vi "iHR550 Correct Center.vi"(1 "Set?":bool=TRUE, 2 "Grating Index":i32=1, 3 "Position In (nm)":dbl=897.9988) -> (0 "Position Out (nm)":dbl=897.9988)   [LabVIEW 2010]
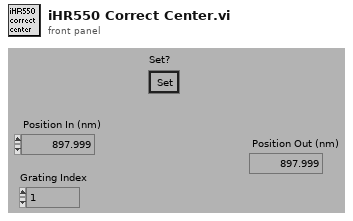
[diagram p1: front panel]
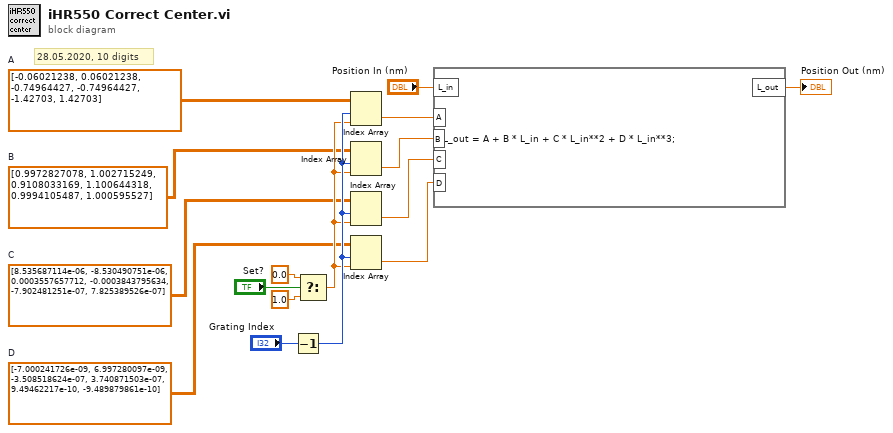
[diagram p0: block diagram]
diagram:
  w1 = dbl[][] [[-7.000241726e-09, 6.997280097e-09], [-3.508518624e-07, 3.740871503e-07], [9.49462217e-10, -9.489879861e-10]]  # D
  w2 = dbl[][] [[8.535687114e-06, -8.530490751e-06], [0.0003557657712, -0.0003843795634], [-7.902481251e-07, 7.825389526e-07]]  # C
  w3 = dbl[][] [[0.9972827078, 1.002715249], [0.9108033169, 1.100644318], [0.9994105487, 1.000595527]]  # B
  w4 = dbl[][] [[-0.06021238, 0.06021238], [-0.74964427, -0.74964427], [-1.42703, 1.42703]]  # A
  # "28.05.2020, 10 digits"
  n1 = Decrement(x="Grating Index") -> (x-1=w15:i32)
  n2 = Select(t=0.0, s="Set?", f=1.0) -> (s? t:f=w11:dbl)
  n3 = Index Array(array=w4, index (row)=w15, index (col)=w11) -> (element=w8:dbl)
  n4 = Index Array(array=w3, index (row)=w15, index (col)=w11) -> (element=w7:dbl)
  n5 = Index Array(array=w2, index (row)=w15, index (col)=w11) -> (element=w6:dbl)
  n6 = Index Array(array=w1, index (row)=w15, index (col)=w11) -> (element=w5:dbl)
  n7 = formula code="L_out = A + B * L_in + C * L_in**2 + D * L_in**3;"("L_in"="Position In (nm)", "A"=w8, "B"=w7, "C"=w6, "D"=w5) -> ("L_out"=→"Position Out (nm)":dbl)
